vi "Load Default Settings.vi"(8 "error in (no error)":errorcluster, 11 "Application in":refnum<class "Application.lvclass">) -> (0 "error out":errorcluster, 3 "Application out":refnum<class "Application.lvclass">)   [LabVIEW 2018, in "Application.lvlib" / "Application.lvclass"]
uses:
  Application.lvclass
  Application.lvclass/Application.ctl
  <vilib>/Utility/xml.llb/Read From XML File(string).vi
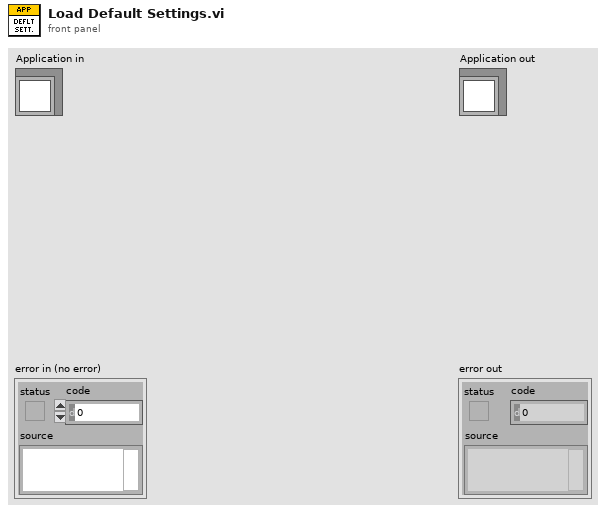
[diagram p1: front panel]
types:
  T1 = typedef "Default Settings.ctl" = cluster{"Refresh Timeout (ms)":i32, "Version String":string, "Hardware Configuration File":string}
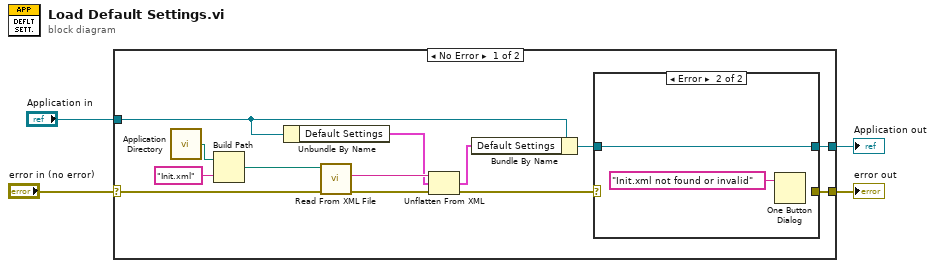
[diagram p0: block diagram]
diagram:
  n1 = case shown="No Error" "error in (no error)" {
    selector: "error in (no error)" -> [w11 w23]
    tunnel: [w7 w23] -> w3
    tunnel: [w5 w22] -> w1
    tunnel: "Application in" -> [w13 w22]
    frame No Error {
      n2 = call <vilib>:"Application Directory.vi"() -> ("Application Directory"=w9:path)
      n3 = Build Path(base path=w9, name or relative path="Init.xml") -> (appended path=w16:path)
      n4 = Unbundle By Name(w13) -> ("Default Settings"=w14:T1)
      n5 = call-poly <vilib>:"Read From XML File.vi"("error in (no error)"=w11, "XML File Path"=w16) -> ("error out"=w10:errorcluster, "XML Elements"=w15:string)  [unwired: 7 in, 1 out]
      n6 = Unflatten From XML(xml string=w15, type=w14, error in (no error)=w10) -> (value=w12:T1, error out=w8:errorcluster)
      n7 = Bundle By Name(cluster=w13, "Default Settings"=w12) -> (w6:refnum<class "Application.lvclass">)
      n8 = case shown="Error" w8 {
        selector: w8 -> [w19 _]
        tunnel: [w19 _] -> w7
        tunnel: w6 -> [w18 w21]
        tunnel: [w18 w21] -> w5
        frame No Error {
        }
        frame Error {
          n9 = One Button Dialog(message="Init.xml not found or invalid") -> ()  [unwired: 1 in, 1 out]
        }
      }
    }
    frame Error {
    }
  }
  "error out" <- w3
  "Application out" <- w1
